vi "Variant to 2D String.vi"(8 "error in (no error)":errorcluster, 10 "Variant":variant[][](array[variant])=[[variant(string "id"), variant(string "int(11)"), variant(string "NO"), variant(string "PRI"), variant(string "\u000eauto_increment"), variant], [variant(string "department_name"), variant(string "varchar(50)"), variant(string "NO"), variant(string ""), variant(string "\u0000"), variant], [variant(string "line_id"), variant(string "int(11)"), variant(string "NO"), variant(string "MUL"), variant(string "\u0000"), variant], [variant(string "status"), variant(string "tinyint(1)"), variant(string "NO"), variant(string ""), variant(string "1"), variant(string "")], [variant(string "mark_data"), variant(string "tinyint(1)"), variant(string "NO"), variant(string ""), variant(string "0"), variant(string "")]]) -> (0 "error out":errorcluster, 2 "2D String":string[][](array[string]))   [LabVIEW 2020]
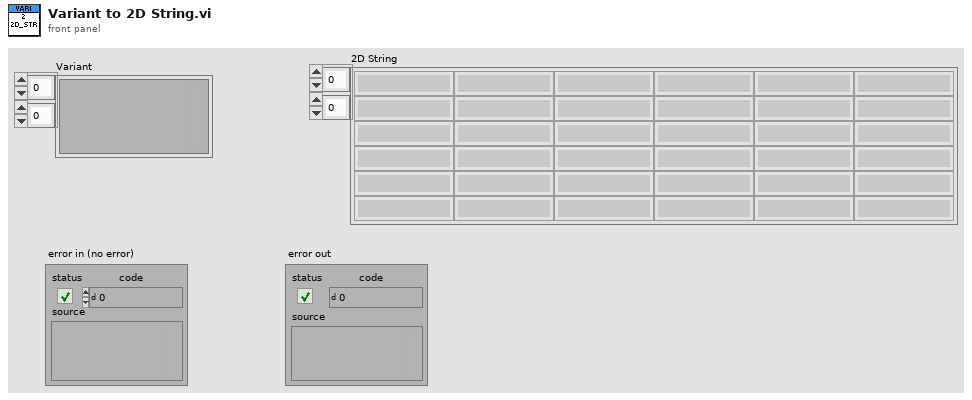
[diagram p1: front panel]
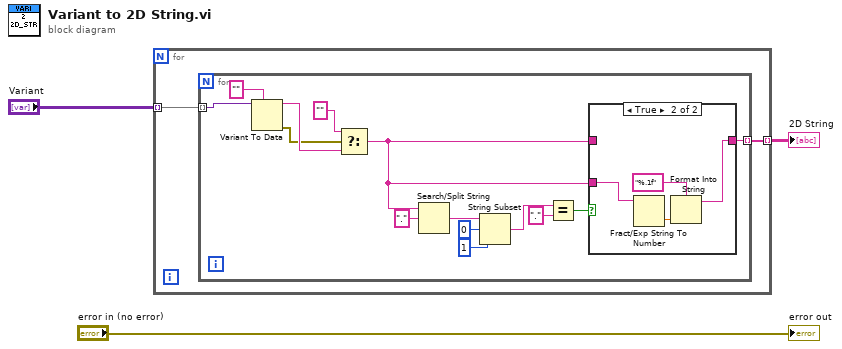
[diagram p0: block diagram]
diagram:
  n1 = for {
    tunnel: "Variant" -> [w5] mode=indexing
    tunnel: [w4] -> w2 mode=indexing
    n2 = for {
      tunnel: w5 -> [w19] mode=indexing
      tunnel: [w12] -> w4 mode=indexing
      n3 = Variant To Data(type="", Variant=w19) -> (data=w16:string, error out=w15:errorcluster)  [unwired: 1 in]
      n4 = Select(t="", s=w15, f=w16) -> (s? t:f=w11:string)
      n5 = Search/Split String(string=w11, search string/char (-)=".") -> (match + rest of string=w7:string)  [unwired: 1 in, 2 out]
      n6 = String Subset(string=w7, offset (0)=0, length (rest)=1 ("length (rest)")) -> (substring=w6:string)
      n7 = Equal?(x=w6, y=".") -> (x = y?=w13:bool)
      n8 = case shown="True" w13 {
        tunnel: w11 -> [_ w24]
        tunnel: w11 -> [w20 _]
        tunnel: [w20 w21] -> w12
        frame False {
        }
        frame True {
          n9 = Fract/Exp String To Number(string=w24) -> (number=w22:dbl)  [unwired: 3 in, 1 out]
          n10 = Format Into String(format string="%.1f", w22) -> (resulting string=w21:string)  [unwired: 2 in, 1 out]
        }
      }
    }
  }
  "2D String" <- w2
  "error out" <- "error in (no error)"
